vi "ADCP_UI_Update_Transmit_List_Table.vi"(8 "error in (no error)":errorcluster, 11 "ADCU_GUI References":T2) -> ()   [LabVIEW 2017]
uses:
  Controls/ADCP_UI/ADCP_UI_Parameters.ctl
  Controls/ADCP_UI/ADCP_UI_Queues.ctl
  Controls/ADCP_UI/ADCP_UI_Continuous_Receiver_States.ctl
  Controls/ADCP_UI/ADCP_Queue_Receive_Log_Queue_Element.ctl
  Controls/Packet/Packet.ctl
  Controls/Packet/Packet_Direction.ctl
  Controls/Packet/Packet_Type.ctl
  Controls/Packet/Packet_Priority.ctl
  Controls/Data Packets/Data_Packet.ctl
  Controls/Data Packets/Parameter.ctl
  Controls/Data Packets/Parameter_Data_Type.ctl
  Controls/Data Packets/Data_Packet_Transmit_Mode.ctl
  <vilib>/Utility/miscctls.llb/LVRowAndColumnTypeDef.ctl
  Controls/Data Packets/Data_Packet_FGV_Commands.ctl
panel:
  out "Last Edit Position":T1
  out "Edit Position":T1
  out "NewVal":T1
  out "Active Cell":T1
  out "Transmit List Table":string[][](table)
  out "Exit":bool
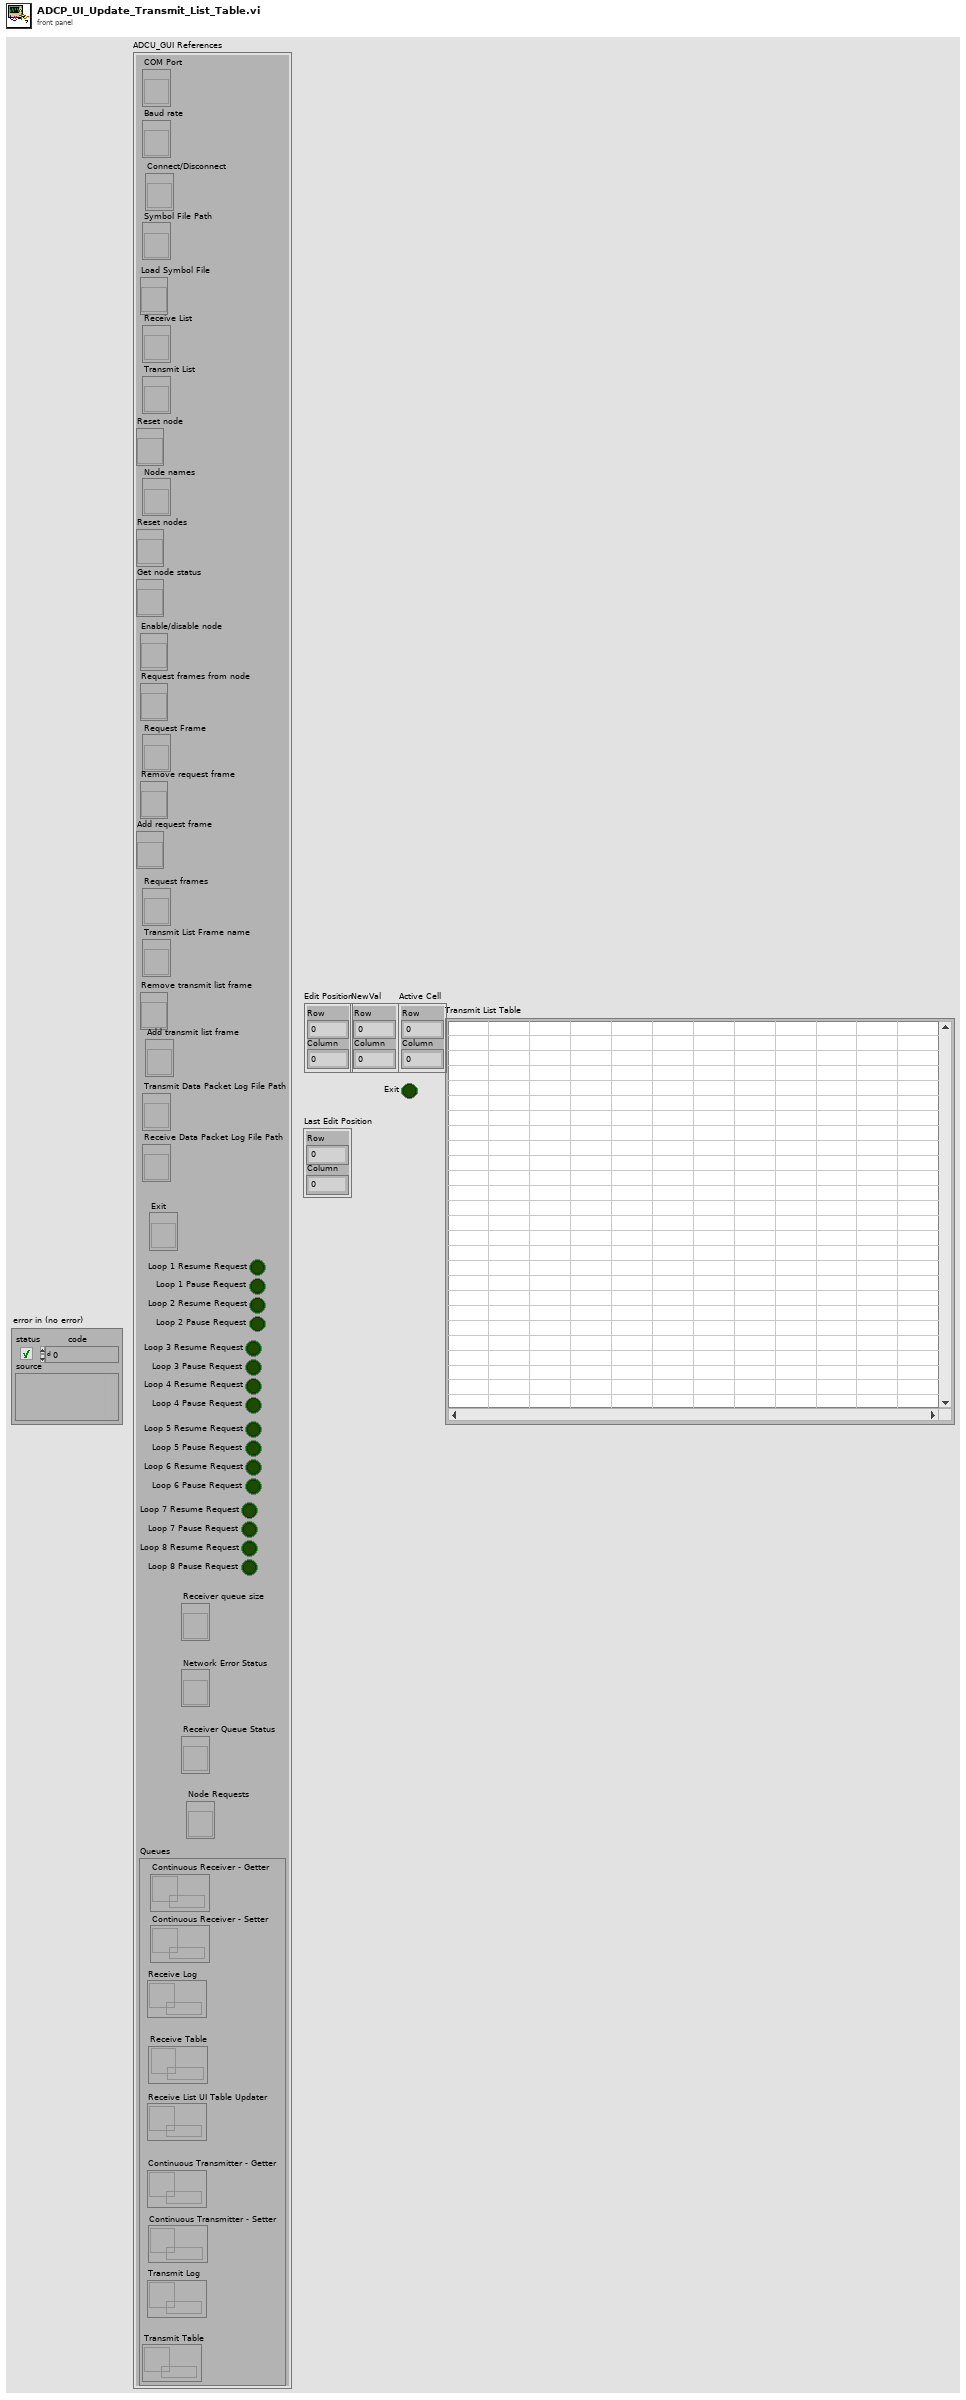
[diagram p1: front panel]
types:
  T1 = typedef "LVRowAndColumnTypeDef.ctl" = cluster{"Row":i32, "Column":i32}
  T2 = typedef "ADCP_UI_Parameters.ctl" = cluster{"COM Port":refnum<vi>, "Baud rate":refnum<vi>, "Symbol File Path":refnum<vi>, "Receive List":refnum<vi>, "Transmit List":refnum<vi>, "Node names":refnum<vi>, "Request Frame":refnum<vi>, "Request frames":refnum<vi>, "Transmit List Frame name":refnum<vi>, "Transmit Data Packet Log File Path":refnum<vi>, "Receive Data Packet Log File Path":refnum<vi>, "Loop 1 Resume Request":bool, "Loop 1 Pause Request":bool, "Loop 2 Resume Request":bool, "Loop 2 Pause Request":bool, "Loop 3 Resume Request":bool, "Loop 3 Pause Request":bool, "Loop 4 Resume Request":bool, "Loop 4 Pause Request":bool, "Loop 5 Resume Request":bool, "Loop 5 Pause Request":bool, "Loop 6 Resume Request":bool, "Loop 6 Pause Request":bool, "Loop 7 Resume Request":bool, "Loop 7 Pause Request":bool, "Loop 8 Resume Request":bool, "Loop 8 Pause Request":bool, "Exit":refnum<vi>, "Connect/Disconnect":refnum<vi>, "Load Symbol File":refnum<vi>, "Reset node":refnum<vi>, "Reset nodes":refnum<vi>, "Get node status":refnum<vi>, "Enable/disable node":refnum<vi>, "Request frames from node":refnum<vi>, "Remove request frame":refnum<vi>, "Add request frame":refnum<vi>, "Remove transmit list frame":refnum<vi>, "Add transmit list frame":refnum<vi>, "Receiver queue size":refnum<vi>, "Network Error Status":refnum<vi>, "Receiver Queue Status":refnum<vi>, "Node Requests":refnum<vi>, "Queues":T3}
  T3 = typedef "ADCP_UI_Queues.ctl" = cluster{"Continuous Receiver - Getter":refnum<queue>, "Continuous Receiver - Setter":refnum<queue>, "Receive Log":refnum<queue>, "Receive Table":refnum<queue>, "Receive List UI Table Updater":refnum<queue>, "Continuous Transmitter - Getter":refnum<queue>, "Continuous Transmitter - Setter":refnum<queue>, "Transmit Log":refnum<queue>, "Transmit Table":refnum<queue>}
  T4 = typedef "Packet_Direction.ctl" = enum16{"Transmit", "Receive", "Bidirectional"}
  T5 = typedef "Data_Packet_FGV_Commands.ctl" = enum16{"Update all parameters from data packets", "Update Packet", "Load", "Read Packet Parameters", "Write Packet Parameters", "Read Packet Parameter", "Write Packet Parameter", "Read Data Packets", "Read Data Packet", "Read Data Packet by Parameter Name", "Get Parameter Node and Frame ID", "Read Data Packet from Node ID and Frame ID"}
  T6 = typedef "Data_Packet_Transmit_Mode.ctl" = enum16{"Disabled", "Single", "Cyclic"}
  T7 = typedef "LVComboBoxStrsAndValuesArrayTypeDef.ctl" = cluster{"String":string, "Value":string}[]
  T8 = typedef "Data_Packet.ctl" = cluster{"Packet":T9, "Parameters":T12[], "Last Received Time (ms)":u64, "Receive count":i32, "Transmit count":i32, "Transmit interval (ms)":u32, "Last Transmitted Time (ms)":u64, "Receive interval (ms)":u32, "Transmit_Mode":T6, "Transmit Enable":bool, "Cyclic Transmit interval (ms)":u32}
  T9 = typedef "Packet.ctl" = cluster{"Raw Bytes":u8[], "Checksum":bool, "Direction":T4, "Processed Bytes":u8[], "Node ID":u8, "Packet type":T10, "Frame Data":u32, "Priority":T11, "Frame ID":u8}
  T10 = typedef "Packet_Type.ctl" = enum16{"Data", "Connection Management", "Remote Request", "Error/Status"}
  T11 = typedef "Packet_Priority.ctl" = enum16{"LOW", "HIGH"}
  T12 = typedef "Parameter.ctl" = cluster{"Parameter name":string, "Node name":string, "Node ID":u8, "Frame name":string, "Frame ID":u8, "Data type":T13, "Start Bit":i32, "Bit Length":i32, "Factor":dbl, "Offset":dbl, "Minimum":dbl, "Maximum":dbl, "Descriptor":string, "Enum values":string[], "Value":string}
  T13 = typedef "Parameter_Data_Type.ctl" = enum16{"BOOL", "UNSIGNED", "SIGNED", "FLOAT32", "ENUM"}
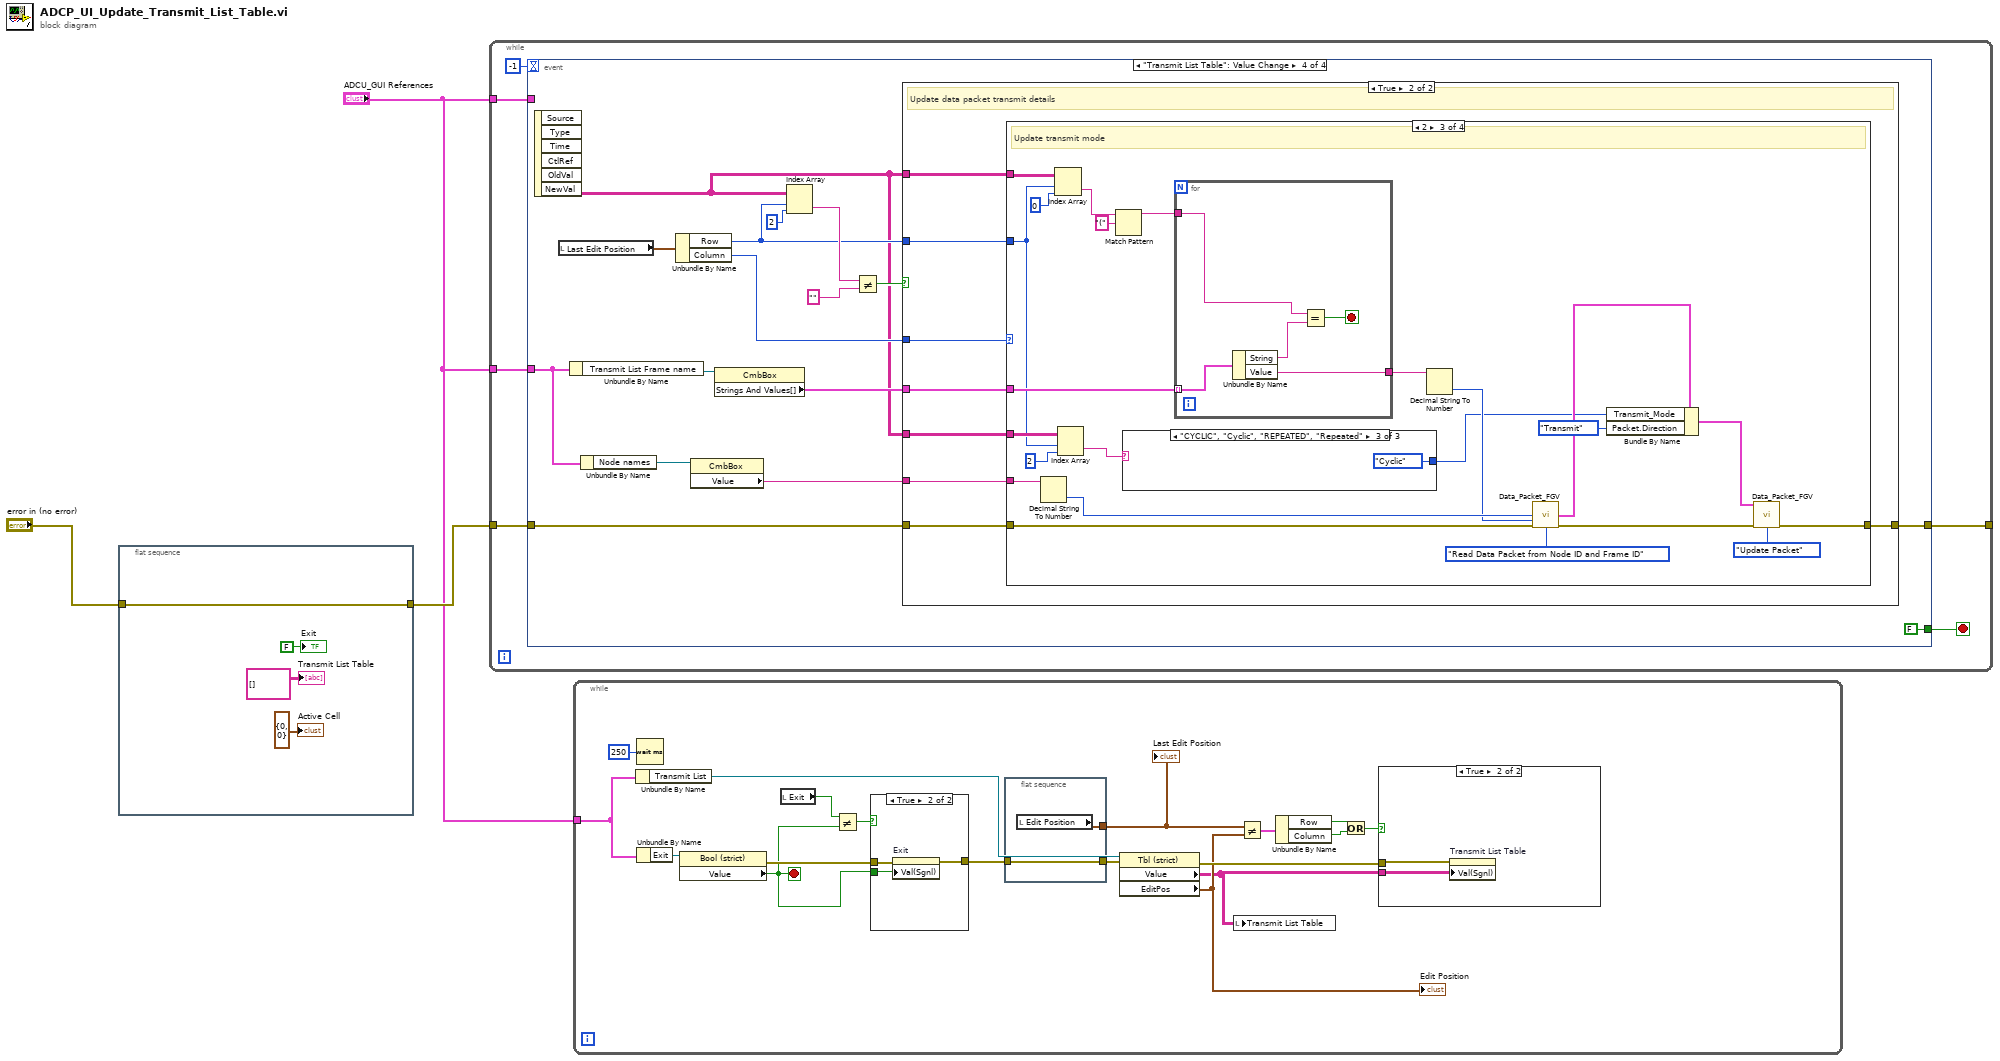
[diagram p0: block diagram]
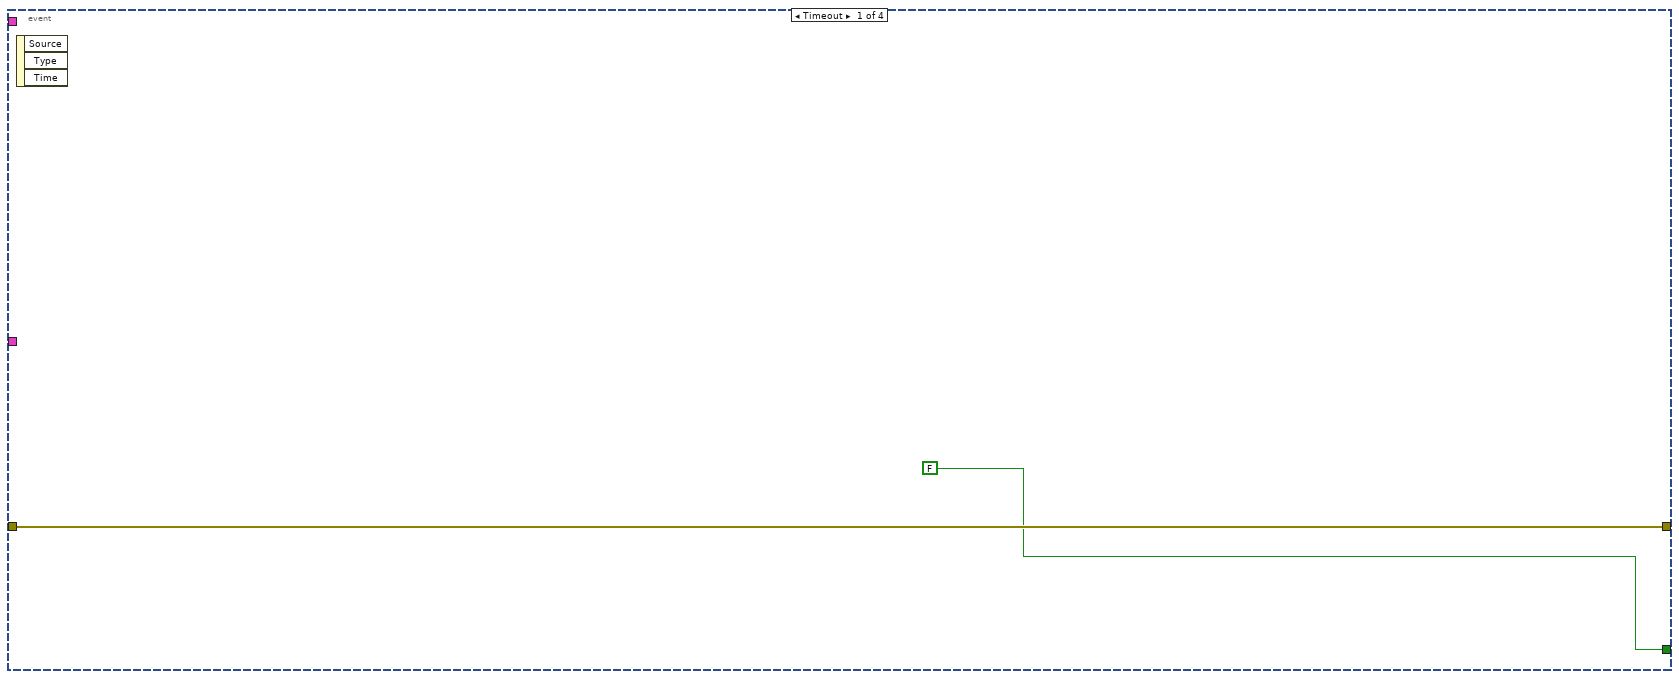
[diagram p4: hidden frame]
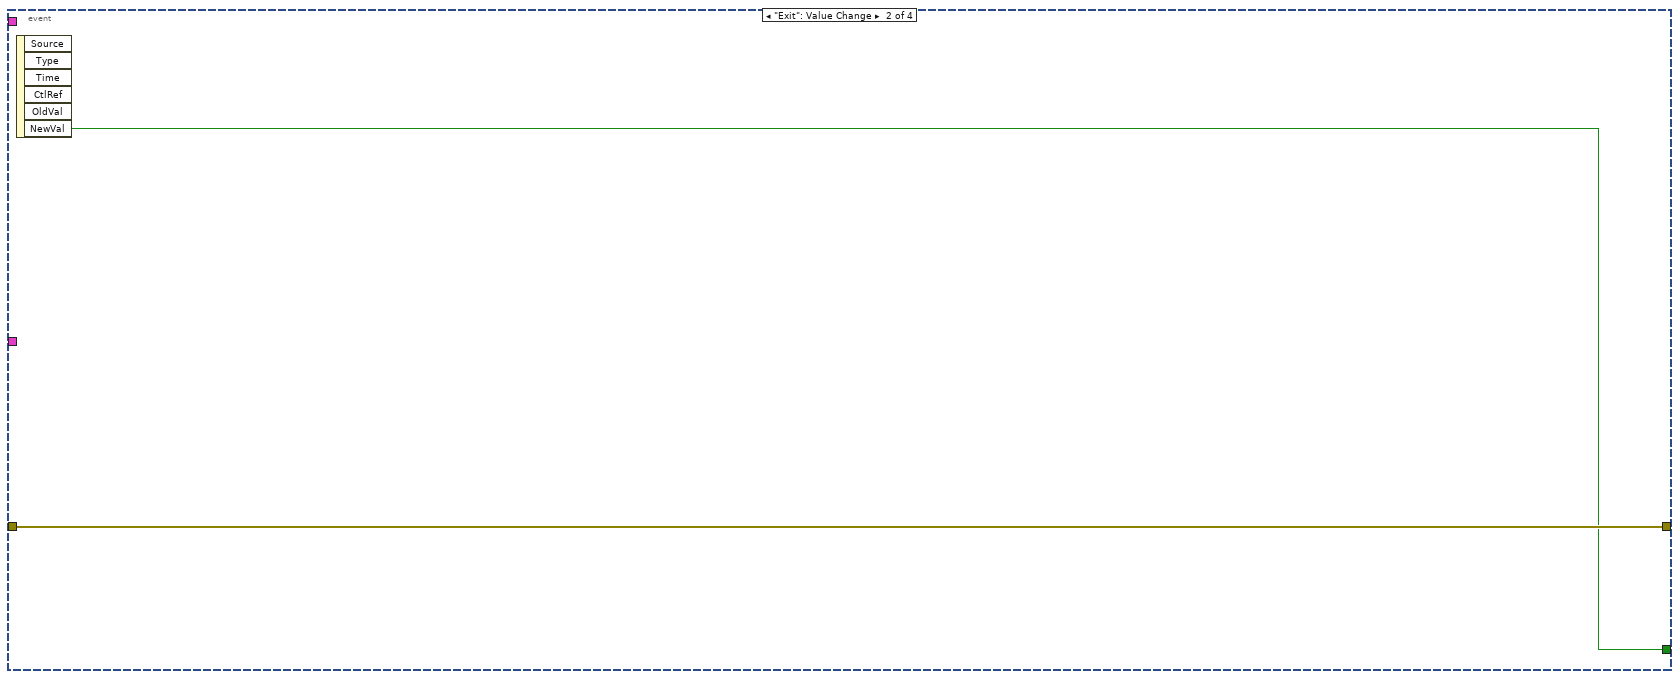
[diagram p5: hidden frame]
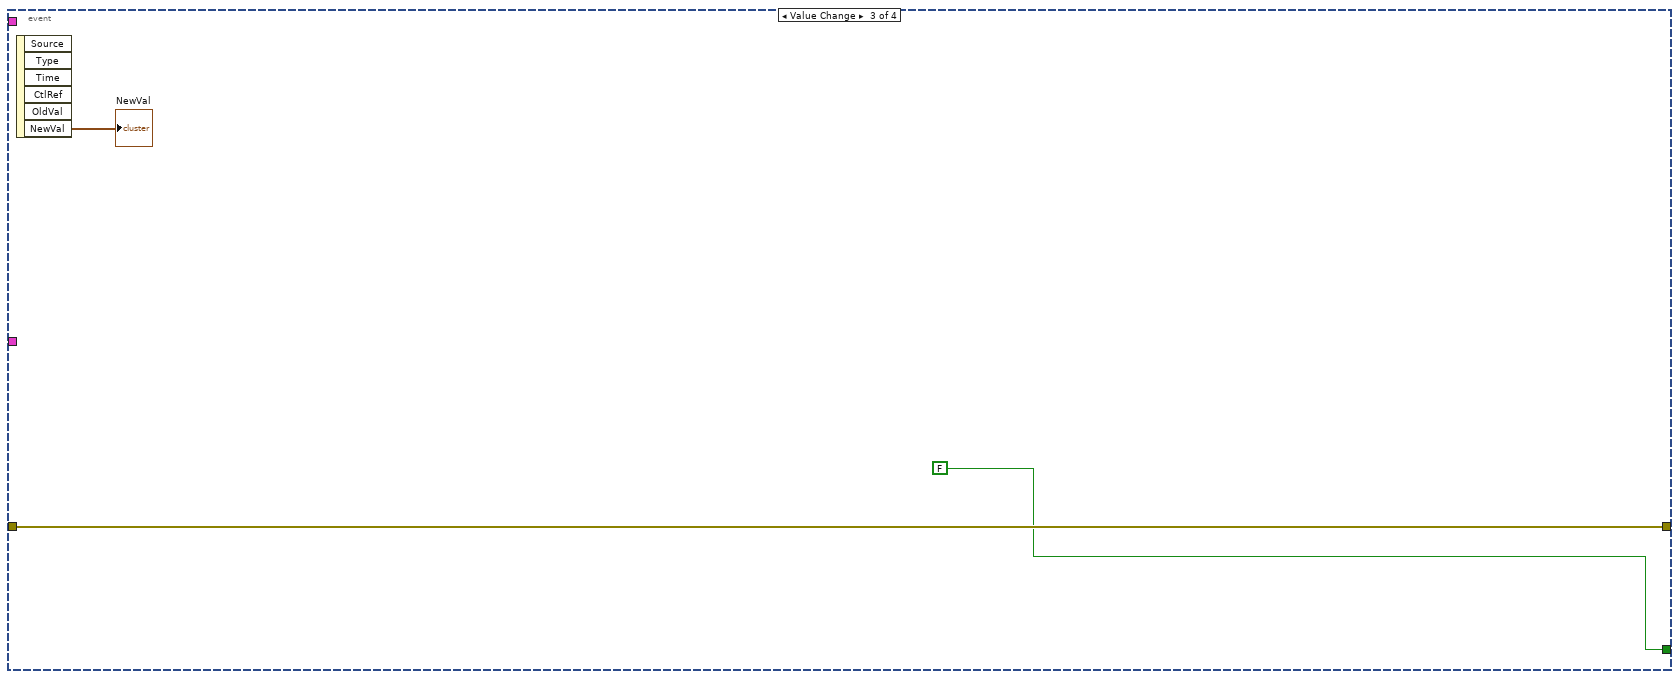
[diagram p6: hidden frame]
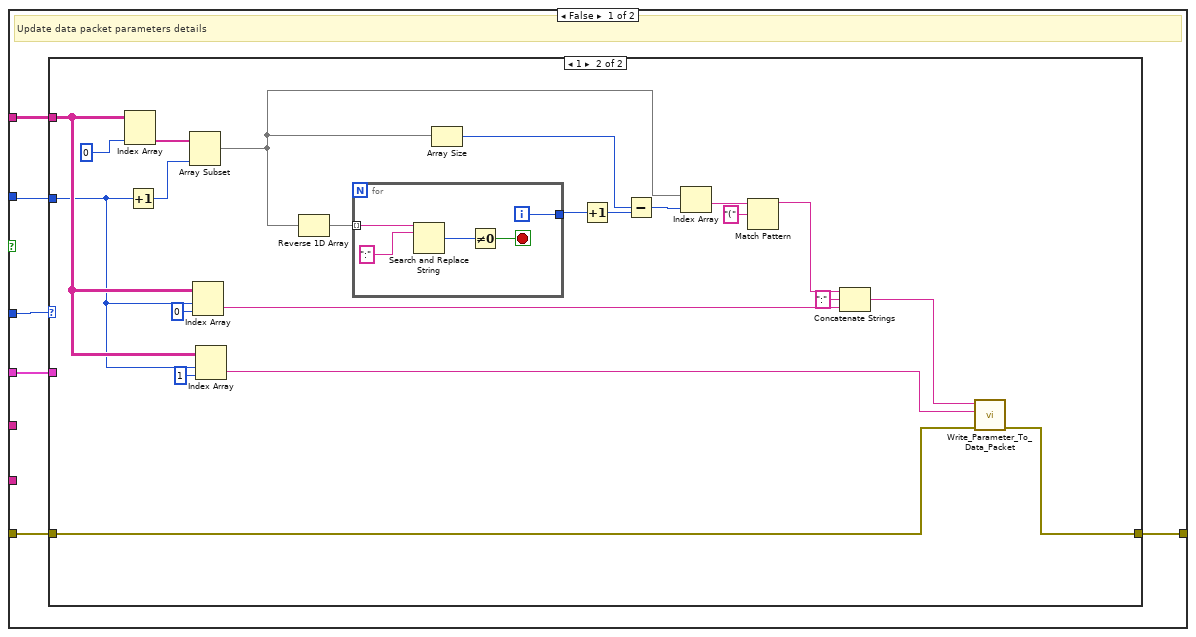
[diagram p7: hidden frame]
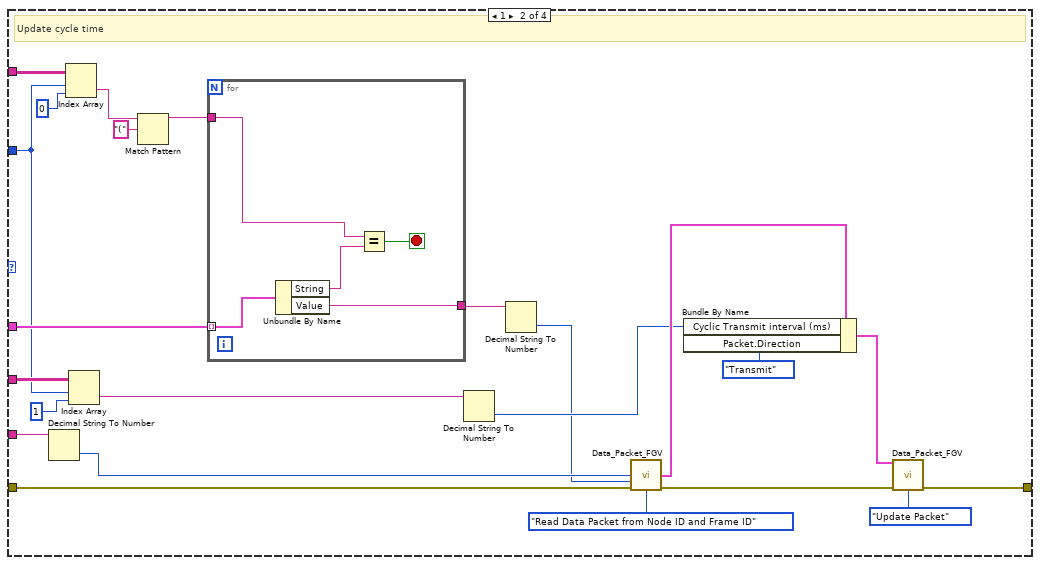
[diagram p10: hidden frame]
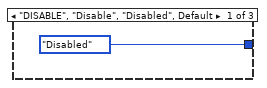
[diagram p11: hidden frame]
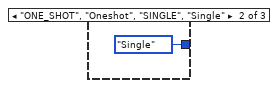
[diagram p12: hidden frame]
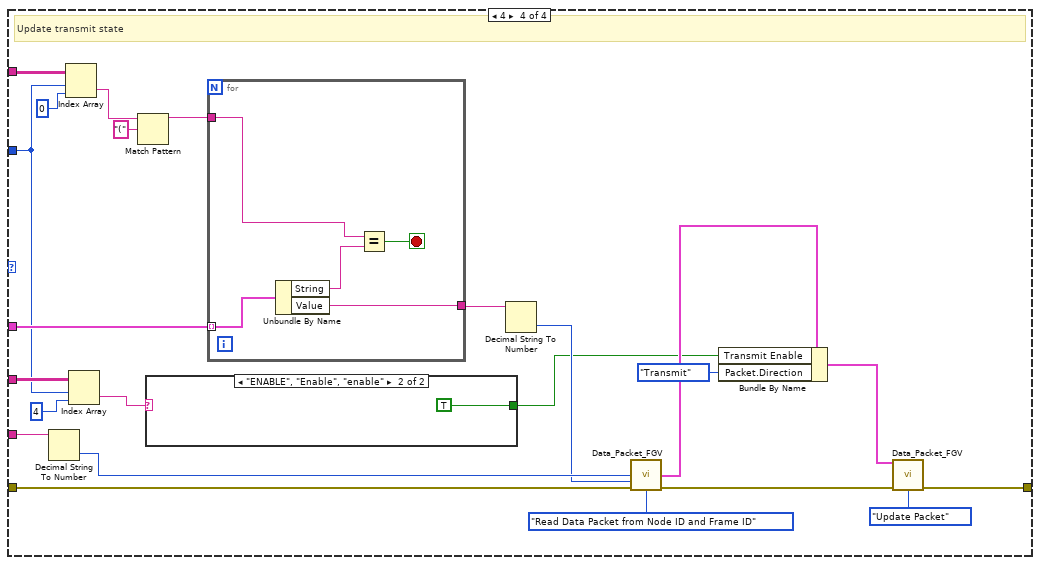
[diagram p13: hidden frame]
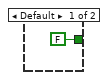
[diagram p14: hidden frame]
diagram:
  n1 = flat-sequence {
    tunnel: "error in (no error)" -> [w7]
    tunnel: [w7] -> w2
    frame #0 {
      "Exit" <- FALSE ("Exit")
      "Transmit List Table" <- string[][] [] ("Transmit List Table")
      "Active Cell" <- T1 {"Row"=0, "Column"=0} ("Active Cell")
    }
  }
  n2 = while {
    tunnel: w2 -> [w13]
    tunnel: "ADCU_GUI References" -> [w12]
    tunnel: [w11] -> _
    tunnel: "ADCU_GUI References" -> [w9]
    stop <- w10 stop-if-true
    n3 = event shown="[3] \"Transmit List Table\": Value Change" {
      selector: _ -> [_ _ _ _]
      dyn-events: _ -> [_ _ _ _]
      timeout: -1 -> [_ _ _ _]
      tunnel: w13 -> [w15 w17 w20 w31]
      tunnel: w12 -> [_ _ _ _]
      tunnel: [w15 w17 w20 w30] -> w11
      tunnel: [FALSE w16 FALSE FALSE ("NewVal")] -> w10
      tunnel: w9 -> [_ _ _ w24]
      event Timeout {
        n4 = event-data() -> ()  [unwired: 1 in, 3 out]
      }
      event "Exit": Value Change {
        n5 = event-data() -> ("NewVal"=w16:bool)  [unwired: 1 in, 5 out]
      }
      event Value Change {
        n6 = event-data() -> ("NewVal"=→"NewVal":T1)  [unwired: 1 in, 5 out]
      }
      event "Transmit List Table": Value Change {
        n7 = event-data() -> ("NewVal"=w21:string[][])  [unwired: 1 in, 5 out]
        n8 = local read "Last Edit Position"() -> (w35:T1)
        n9 = Unbundle By Name(w24) -> ("Transmit List Frame name"=w26:refnum<vi>)
        n10 = Unbundle By Name(w24) -> ("Node names"=w23:refnum<vi>)
        n11 = Unbundle By Name(w35) -> ("Row"=w27:i32, "Column"=w28:i32)
        n12 = property class="CmbBox"(reference=w23) -> ("Value"=w22:string)  [unwired: 1 in, 2 out]
        n13 = property class="CmbBox"(reference=w26) -> ("Strings And Values[]"=w25:T7)  [unwired: 1 in, 2 out]
        n14 = Index Array(array=w21, index (row)=w27, index (col)=2 ("disabled index (col)")) -> (element=w33:string)
        n15 = Not Equal?(x=w33, y="") -> (x != y?=w29:bool)
        n16 = case shown="True" w29 {
          tunnel: w31 -> [w42 w78]
          tunnel: [w41 w77] -> w30
          tunnel: w28 -> [w39 w76]
          tunnel: w21 -> [w40 w75]
          tunnel: w27 -> [w38 w74]
          tunnel: w25 -> [w37 w73]
          tunnel: w22 -> [_ w72]
          tunnel: w21 -> [_ w71]
          frame False {
            # "Update data packet parameters details"
            n17 = case shown="1" w39 {
              tunnel: w42 -> [w43 w46]
              tunnel: [w43 w45] -> w41
              tunnel: w40 -> [_ w50]
              tunnel: w38 -> [_ w49]
              tunnel: w37 -> [_ _]
              frame Default {
              }
              frame 1 {
                n18 = Index Array(array=w50, index (col)=0 ("disabled index (col)")) -> (element=w59:string[])  [unwired: 1 in]
                n19 = Increment(x=w49) -> (x+1=w58:i32)
                n20 = Array Subset(array=w59, length=w58) -> (w57:string[])  [unwired: 1 in]
                n21 = Index Array(array=w50, index (row)=w49, index (col)=0 ("disabled index (col)")) -> (element=w53:string)
                n22 = Index Array(array=w50, index (row)=w49, index (col)=1 ("disabled index (col)")) -> (element=w47:string)
                n23 = Reverse 1D Array(array=w57) -> (reversed array=w64:string[])
                n24 = for {
                  tunnel: w64 -> [w70] mode=indexing
                  tunnel: [w66] -> w63
                  i -> [w66]
                  stop <- w67 stop-if-true
                  n25 = Search and Replace String(input string=w70, search string=":") -> (number of replacements=w68:i32)  [unwired: 6 in, 3 out]
                  n26 = Not Equal To 0?(x=w68) -> (x != 0?=w67:bool)
                }
                n27 = Array Size(array=w57) -> (size(s)=w62:i32)
                n28 = Increment(x=w63) -> (x+1=w60:i32)
                n29 = Subtract(x=w62, y=w60) -> (x-y=w61:i32)
                n30 = Index Array(array=w57, index=w61) -> (element=w56:string)
                n31 = Match Pattern(string=w56, regular expression="(") -> (before substring=w44:string)  [unwired: 1 in, 3 out]
                n32 = Concatenate Strings(w44, ":" ("string"), w53) -> (w52:string)
                n33 = call "Write_Parameter_To_Data_Packet.vi"("error in (no error)"=w46, "Parameter value"=w47, "Parameter name"=w52) -> ("error out"=w45:errorcluster)  [unwired: 7 in, 1 out]
              }
            }
          }
          frame True {
            # "Update data packet transmit details"
            n34 = case shown="2" w76 {
              tunnel: w78 -> [w79 w94 w122 w153]
              tunnel: [w79 w83 w113 w144] -> w77
              tunnel: w75 -> [_ w102 w130 w161]
              tunnel: w74 -> [_ w90 w118 w149]
              tunnel: w73 -> [_ w98 w126 w157]
              tunnel: w72 -> [_ w95 w123 w154]
              tunnel: w71 -> [_ w91 w119 w150]
              frame Default {
              }
              frame 1 {
                # "Update cycle time"
                n35 = Decimal String To Number(string=w95) -> (number=w86:i32)  [unwired: 2 in, 1 out]
                n36 = Index Array(array=w102, index (row)=w90, index (col)=0 ("disabled index (col)")) -> (element=w100:string)
                n37 = Index Array(array=w91, index (row)=w90, index (col)=1 ("disabled index (col)")) -> (element=w88:string)
                n38 = Match Pattern(string=w100, regular expression="(") -> (before substring=w97:string)  [unwired: 1 in, 3 out]
                n39 = for {
                  tunnel: w98 -> [w106] mode=indexing
                  tunnel: w97 -> [w107]
                  tunnel: [w104] -> w96
                  stop <- w103 stop-if-true
                  n40 = Unbundle By Name(w106) -> ("String"=w105:string, "Value"=w104:string)
                  n41 = Equal?(x=w107, y=w105) -> (x = y?=w103:bool)
                }
                n42 = Decimal String To Number(string=w88) -> (number=w87:i32)  [unwired: 2 in, 1 out]
                n43 = Decimal String To Number(string=w96) -> (number=w85:i32)  [unwired: 2 in, 1 out]
                n44 = call "Data_Packet_FGV.vi"("Node ID"=w86, "Frame ID"=w85, "error in (no error)"=w94, "Commands"=Data_Packet_FGV_Commands."Read Data Packet from Node ID and Frame ID") -> ("Data_Packet out"=w92:T8, "error out"=w84:errorcluster)  [unwired: 6 in, 4 out]
                n45 = Bundle By Name(cluster=w92, "Cyclic Transmit interval (ms)"=w87, "Packet.Direction"=Packet_Direction."Transmit") -> (w82:T8)
                n46 = call "Data_Packet_FGV.vi"("Data_Packet In"=w82, "error in (no error)"=w84, "Commands"=Data_Packet_FGV_Commands."Update Packet") -> ("error out"=w83:errorcluster)  [unwired: 7 in, 5 out]
              }
              frame 2 {
                # "Update transmit mode"
                n47 = Decimal String To Number(string=w123) -> (number=w116:i32)  [unwired: 2 in, 1 out]
                n48 = Index Array(array=w130, index (row)=w118, index (col)=0 ("disabled index (col)")) -> (element=w128:string)
                n49 = Index Array(array=w119, index (row)=w118, index (col)=2 ("disabled index (col)")) -> (element=w110:string)
                n50 = Match Pattern(string=w128, regular expression="(") -> (before substring=w125:string)  [unwired: 1 in, 3 out]
                n51 = case shown="\"CYCLIC\", \"Cyclic\", \"REPEATED\", \"Repeated\"" w110 {
                  tunnel: [Data_Packet_Transmit_Mode."Disabled" ("Transmit_Mode") Data_Packet_Transmit_Mode."Single" ("Transmit_Mode") Data_Packet_Transmit_Mode."Cyclic" ("Transmit_Mode")] -> w109
                  frame "DISABLE", "Disable", "Disabled", Default {
                  }
                  frame "ONE_SHOT", "Oneshot", "SINGLE", "Single" {
                  }
                  frame "CYCLIC", "Cyclic", "REPEATED", "Repeated" {
                  }
                }
                n52 = for {
                  tunnel: w126 -> [w137] mode=indexing
                  tunnel: w125 -> [w138]
                  tunnel: [w135] -> w124
                  stop <- w134 stop-if-true
                  n53 = Unbundle By Name(w137) -> ("String"=w136:string, "Value"=w135:string)
                  n54 = Equal?(x=w138, y=w136) -> (x = y?=w134:bool)
                }
                n55 = Decimal String To Number(string=w124) -> (number=w115:i32)  [unwired: 2 in, 1 out]
                n56 = call "Data_Packet_FGV.vi"("Node ID"=w116, "Frame ID"=w115, "error in (no error)"=w122, "Commands"=Data_Packet_FGV_Commands."Read Data Packet from Node ID and Frame ID") -> ("Data_Packet out"=w120:T8, "error out"=w114:errorcluster)  [unwired: 6 in, 4 out]
                n57 = Bundle By Name(cluster=w120, "Transmit_Mode"=w109, "Packet.Direction"=Packet_Direction."Transmit") -> (w112:T8)
                n58 = call "Data_Packet_FGV.vi"("Data_Packet In"=w112, "error in (no error)"=w114, "Commands"=Data_Packet_FGV_Commands."Update Packet") -> ("error out"=w113:errorcluster)  [unwired: 7 in, 5 out]
              }
              frame 4 {
                # "Update transmit state"
                n59 = Decimal String To Number(string=w154) -> (number=w147:i32)  [unwired: 2 in, 1 out]
                n60 = Index Array(array=w161, index (row)=w149, index (col)=0 ("disabled index (col)")) -> (element=w159:string)
                n61 = Index Array(array=w150, index (row)=w149, index (col)=4 ("disabled index (col)")) -> (element=w141:string)
                n62 = Match Pattern(string=w159, regular expression="(") -> (before substring=w156:string)  [unwired: 1 in, 3 out]
                n63 = case shown="\"ENABLE\", \"Enable\", \"enable\"" w141 {
                  tunnel: [FALSE TRUE] -> w140
                  frame Default {
                  }
                  frame "ENABLE", "Enable", "enable" {
                  }
                }
                n64 = for {
                  tunnel: w157 -> [w167] mode=indexing
                  tunnel: w156 -> [w168]
                  tunnel: [w165] -> w155
                  stop <- w164 stop-if-true
                  n65 = Unbundle By Name(w167) -> ("String"=w166:string, "Value"=w165:string)
                  n66 = Equal?(x=w168, y=w166) -> (x = y?=w164:bool)
                }
                n67 = Decimal String To Number(string=w155) -> (number=w146:i32)  [unwired: 2 in, 1 out]
                n68 = call "Data_Packet_FGV.vi"("Node ID"=w147, "Frame ID"=w146, "error in (no error)"=w153, "Commands"=Data_Packet_FGV_Commands."Read Data Packet from Node ID and Frame ID") -> ("Data_Packet out"=w151:T8, "error out"=w145:errorcluster)  [unwired: 6 in, 4 out]
                n69 = Bundle By Name(cluster=w151, "Transmit Enable"=w140, "Packet.Direction"=Packet_Direction."Transmit") -> (w143:T8)
                n70 = call "Data_Packet_FGV.vi"("Data_Packet In"=w143, "error in (no error)"=w145, "Commands"=Data_Packet_FGV_Commands."Update Packet") -> ("error out"=w144:errorcluster)  [unwired: 7 in, 5 out]
              }
            }
          }
        }
      }
    }
  }
  n71 = while {
    tunnel: "ADCU_GUI References" -> [w181]
    stop <- w182 stop-if-true
    n72 = Unbundle By Name(w181) -> ("Transmit List"=w179:refnum<vi>)
    n73 = Wait (ms)(milliseconds to wait=u32 250) -> ()  [unwired: 1 out]
    n74 = Unbundle By Name(w181) -> ("Exit"=w186:refnum<vi>)
    n75 = property class="Bool (strict)"(reference=w186) -> (error out=w185:errorcluster, "Value"=w182:bool)  [unwired: 1 in, 1 out]
    n76 = local read "Exit"() -> (w184:bool)
    n77 = Not Equal?(x=w184, y=w182) -> (x != y?=w183:bool)
    n78 = case shown="True" w183 {
      tunnel: w185 -> [w191 w194]
      tunnel: [w191 w193] -> w177
      tunnel: w182 -> [_ w192]
      frame False {
      }
      frame True {
        n79 = property on="Exit" class="Bool (strict)"(error in=w194, "Val(Sgnl)"=w192) -> (error out=w193:errorcluster)  [unwired: 1 in, 1 out]
      }
    }
    n80 = flat-sequence {
      tunnel: w177 -> [w188]
      tunnel: [w188] -> w176
      tunnel: [w187] -> w174
      frame #0 {
        n81 = local read "Edit Position"() -> (w187:T1)
      }
    }
    n82 = property class="Tbl (strict)"(reference=w179, error in=w176) -> (error out=w178:errorcluster, "Value"=w169:string[][], "EditPos"=w175:T1)  [unwired: 1 out]
    "Edit Position" <- w175
    n83 = local write "Transmit List Table"(w169) -> ()
    n84 = Not Equal?(x=w174, y=w175) -> (x != y?=w173:cluster{"Row":bool, "Column":bool})
    n85 = Unbundle By Name(w173) -> ("Row"=w172:bool, "Column"=w171:bool)
    n86 = Or(x=w172, y=w171) -> (x .or. y?=w170:bool)
    n87 = case shown="True" w170 {
      tunnel: w178 -> [_ w190]
      tunnel: w169 -> [_ w189]
      frame False {
      }
      frame True {
        n88 = property on="Transmit List Table" class="Tbl (strict)"(error in=w190, "Val(Sgnl)"=w189) -> ()  [unwired: 1 in, 2 out]
      }
    }
    "Last Edit Position" <- w174
  }
